vi "VI Tree - JKI State Machine.vi"   [LabVIEW 2013]
panel:
  # "VI TREE"
  # "For instructions on how to use the JKI State Machine, examples and video tutorials, visit:\nhttp://jki.net/state-machine/\n\nJKI State Machine™\nhttp://jki.net/state-machine/\nCopyright (C) 2005-2020, JKI <info@jki.net>\nALL RIGHTS RESERVED"
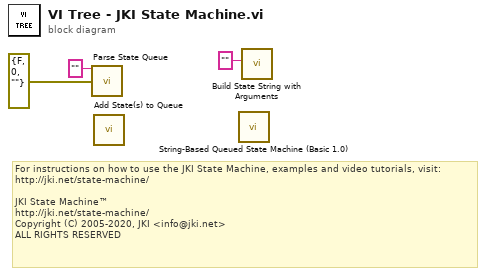
[diagram p0: block diagram]
diagram:
  # "For instructions on how to use the JKI State Machine, examples and video tutorials, visit:\nhttp://jki.net/state-machine/\n\nJKI State Machine™\nhttp://jki.net/state-machine/\nCopyright (C) 2005-2020, JKI <info@jki.net>\nALL RIGHTS RESERVED"
  n1 = call "Parse State Queue.vi"("State Queue"="", "Error In (no error)"=errorcluster {"status"=FALSE, "code"=0, "source"=""} ("Error")) -> ()  [unwired: 11 in, 3 out]
  n2 = call "Add State(s) to Queue.vi"() -> ()  [unwired: 15 in, 1 out]
  n3 = call "String-Based Queued State Machine (Basic 1.0).vi"() -> ()  [unwired: 1 in]
  n4 = call "Build State String with Arguments.vi"("State"="" ("State (\"\")")) -> ()  [unwired: 5 in, 1 out]
